vi "ESP301_Open.vi"(11 "strDeviceKey":string) -> (0 "sortie d'erreur":errorcluster, 3 "référence en sortie":refnum<k24>)   [LabVIEW 2019]
uses:
  Newport.ESP301.CommandInterface
panel:
  out "OpenInstrument":i32
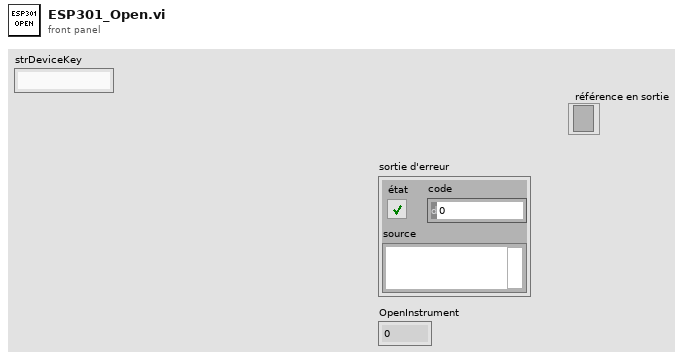
[diagram p1: front panel]
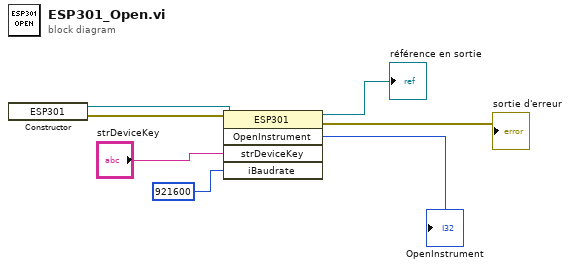
[diagram p0: block diagram]
diagram:
  n1 = constructor class="ESP301"() -> (reference out=w7:refnum<k24>, error out=w6:errorcluster)  [unwired: 3 in, 1 out]
  n2 = invoke on="Nœud de méthode" class="ESP301" method="OpenInstrument"(reference=w7, error in=w6, "strDeviceKey"="strDeviceKey", "iBaudrate"=921600) -> (reference out=→"référence en sortie":refnum<k24>, error out=→"sortie d'erreur":errorcluster, "OpenInstrument"=→"OpenInstrument":i32)  [unwired: 1 in, 2 out]
